vi "Turn Smother.vi"(2 "Ignore Deceleration":bool, 3 "Ignore Acceleration":bool, 4 "input cluster":T5={"Trajectory Data"=[], "Updated Waypoints"=[], "Parameters"={"Sample Period (s)"=0.0, "Limits"={"Velocity (fps)"=6.0, "Accel (fps^2)"=15.0, "Jerk (fps^3)"=150.0, "StoopidFast (fps)"=6.0}, "Conditions"={"vInitial (fps)"=0.0, "vFinal (fps)"=0.0}, "Overrides"=[]}, "Array"=[]} {"Parameters"."Overrides"."Angular Multiplier 2" step=5.0; "Parameters"."Overrides"."Angular Multiplier" step=5.0; "Parameters"."Limits"."StoopidFast (fps)" min=0.0; "Parameters"."Limits"."Jerk (fps^3)" min=0.0 step=1.0; "Parameters"."Limits"."Accel (fps^2)" min=0.0; "Parameters"."Limits"."Velocity (fps)" min=0.0}) -> (1 "Overrides":T1(array[cluster]) {"Angular Multiplier 2" step=5.0; "Angular Multiplier" step=5.0})   [LabVIEW 2019]
uses:
  Types/Limits.ctl
  Types/Single Cmd Info.ctl
  <vilib>/picture/picture.llb/imagedata.ctl
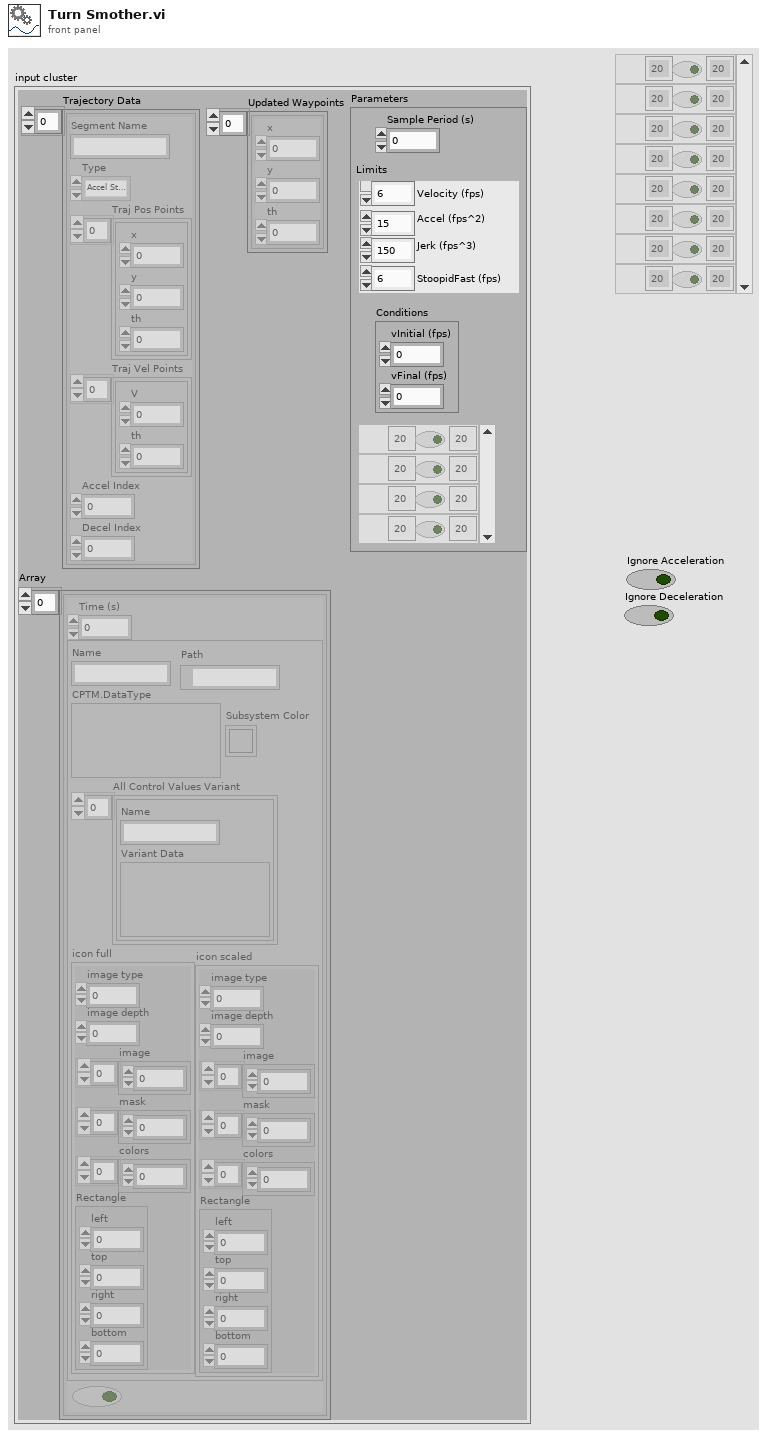
[diagram p1: front panel]
types:
  T1 = cluster{"Count":string, "Angular Multiplier":dbl, "1":bool, "Angular Multiplier 2":dbl}[]
  T2 = typedef "Limits.ctl" = cluster{"Velocity (fps)":dbl, "Accel (fps^2)":dbl, "Jerk (fps^3)":dbl, "StoopidFast (fps)":dbl}
  T3 = typedef "Single Cmd Info.ctl" = cluster{"Name":string, "CPTM.DataType":variant, "All Control Values Variant":cluster{"Name":string, "Variant Data":variant}[], "icon full":T4, "icon scaled":T4, "Path":path, "Subsystem Color":u32}
  T4 = typedef "imagedata.ctl" = cluster{"image type":i32, "image depth":i32, "image":u8[], "mask":u8[], "colors":u32[], "Rectangle":cluster{"left":i16, "top":i16, "right":i16, "bottom":i16}}
  T5 = cluster{"Trajectory Data":cluster{"Segment Name":string, "Type":enum16{"Accel Straight", "Const Straight", "Blend", "Circle"}, "Traj Pos Points":cluster{"x":dbl, "y":dbl, "th":dbl}[], "Traj Vel Points":cluster{"V":dbl, "th":dbl}[], "Accel Index":i32, "Decel Index":i32}[], "Updated Waypoints":cluster{"x":dbl, "y":dbl, "th":dbl}[], "Parameters":cluster{"Sample Period (s)":dbl, "Limits":T2, "Conditions":cluster{"vInitial (fps)":dbl, "vFinal (fps)":dbl}, "Overrides":cluster{"Count":string, "Angular Multiplier":dbl, "1":bool, "Angular Multiplier 2":dbl}[]}, "Array":cluster{"Time (s)":dbl, T3, bool}[]}
  T6 = cluster{"Segment Name":string, "Type":enum16{"Accel Straight", "Const Straight", "Blend", "Circle"}, "Traj Pos Points":cluster{"x":dbl, "y":dbl, "th":dbl}[], "Traj Vel Points":cluster{"V":dbl, "th":dbl}[], "Accel Index":i32, "Decel Index":i32}[]
  T7 = cluster{"Sample Period (s)":dbl, "Limits":T2, "Conditions":cluster{"vInitial (fps)":dbl, "vFinal (fps)":dbl}, "Overrides":cluster{"Count":string, "Angular Multiplier":dbl, "1":bool, "Angular Multiplier 2":dbl}[]}
  T8 = cluster{"vInitial (fps)":dbl, "vFinal (fps)":dbl}
  T9 = cluster{string, dbl, bool, "Velocity (fps)":dbl}[]
  T10 = cluster{"Segment Name":string, "Type":enum16{"Accel Straight", "Const Straight", "Blend", "Circle"}, "Traj Pos Points":cluster{"x":dbl, "y":dbl, "th":dbl}[], "Traj Vel Points":cluster{"V":dbl, "th":dbl}[], "Accel Index":i32, "Decel Index":i32}
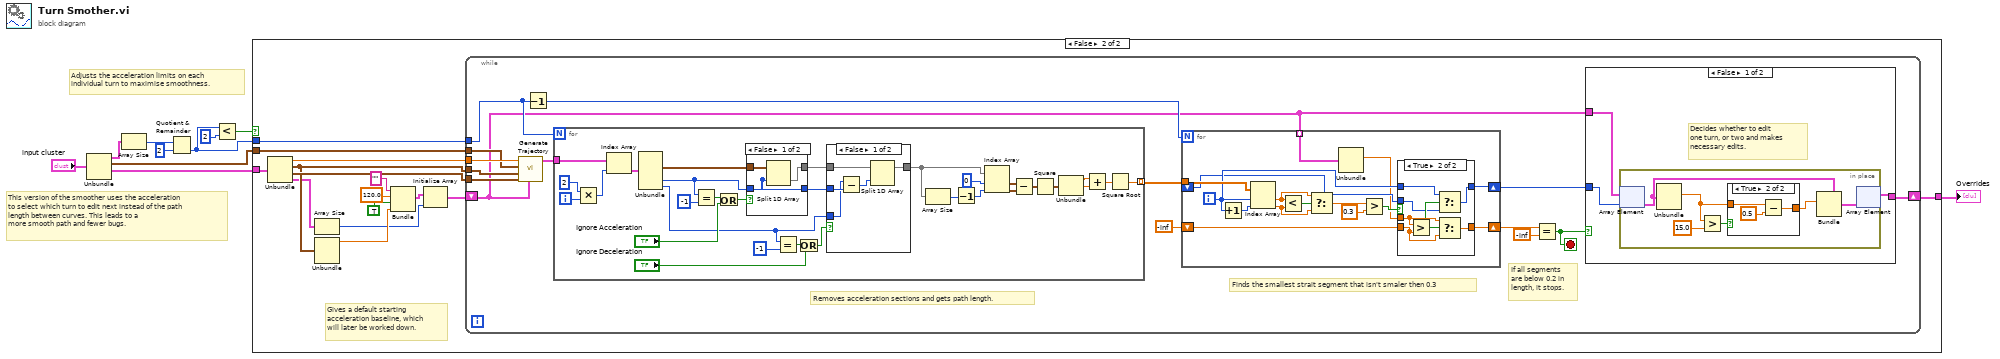
[diagram p0: block diagram]
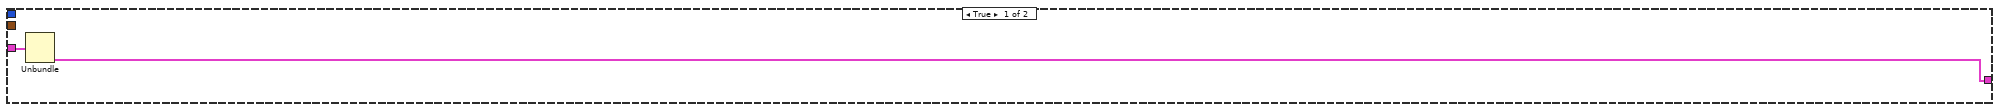
[diagram p2: hidden frame]
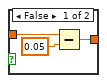
[diagram p3: hidden frame]
diagram:
  # "This version of the smoother uses the acceleration\nto select which turn to edit next instead of the path \nlength between curves. This leads to a \nmore smooth path and fewer bugs."
  # "Adjusts the acceleration limits on each \nindividual turn to maximise smoothness."
  n1 = Unbundle("input cluster") -> ("Trajectory Data"=w3:T6, "Updated Waypoints"=w2:cluster{"x":dbl, "y":dbl, "th":dbl}[], "Parameters"=w4:T7)  [unwired: 1 out]
  n2 = Array Size(array=w3) -> (size(s)=w10:i32)
  n3 = Quotient & Remainder(x=w10, y=2) -> (floor(x/y)=w6:i32)  [unwired: 1 out]
  n4 = Less?(x=w6, y=2) -> (x < y?=w5:bool)
  n5 = case shown="False" w5 {
    tunnel: w6 -> [_ w27]
    tunnel: [w12 w26] -> w1
    tunnel: w4 -> [w11 w25]
    tunnel: w2 -> [_ w23]
    frame True {
      n6 = Unbundle(w11) -> ("Overrides"=w12:T1)  [unwired: 3 out]
    }
    frame False {
      # "Gives a default starting \nacceleration baseline, which\nwill later be worked down."
      n7 = Unbundle(w25) -> ("Sample Period (s)"=w24:dbl, "Limits"=w21:T2, "Conditions"=w22:T8, "Overrides"=w20:T1)
      n8 = Array Size(array=w20) -> (size(s)=w15:i32)
      n9 = Unbundle(w21) -> ("Velocity (fps)"=w16:dbl)  [unwired: 3 out]
      n10 = Bundle("", 120.0, TRUE, "Velocity (fps)"=w16) -> (w14:cluster{string, dbl, bool, "Velocity (fps)":dbl})  [unwired: 1 in]
      n11 = Initialize Array(w14, w15) -> (w13:T9)
      n12 = while {
        shift-right: [w40] -> w26
        shift-left: w13 -> [w28]
        tunnel: w27 -> [w37]
        tunnel: w24 -> [w35]
        tunnel: w23 -> [w34]
        tunnel: w21 -> [w33]
        tunnel: w22 -> [w32]
        stop <- w42 stop-if-true
        # "If all segments\nare below 0.2 in\nlength, it stops."
        # "Removes acceleration sections and gets path length."
        # "Finds the smallest strait segment that isn't smaler then 0.3"
        n13 = call "Generate Trajectory.vi"("Overrides 2"=w28, "Conditions"=w32, "Limits"=w33, "WayPoints"=w34, "Sample Period (s)"=w35) -> ("Trajectory Data"=w36:T6)  [unwired: 2 in, 4 out]
        n14 = Decrement(x=w37) -> (x-1=w38:i32)
        n15 = for {
          N: w37 -> [_]
          tunnel: w36 -> [w86]
          tunnel: [w76] -> w39 mode=indexing
          i -> [w88]
          n16 = Multiply(x=2, y=w88) -> (x*y=w85:i32)
          n17 = Index Array(array=w86, index=w85) -> (element=w84:T10)
          n18 = Unbundle(w84) -> ("Traj Pos Points"=w77:cluster{"x":dbl, "y":dbl, "th":dbl}[], "Accel Index"=w73:i32, "Decel Index"=w66:i32)  [unwired: 3 out]
          n19 = Equal?(x=w73, y=-1) -> (x = y?=w74:bool)
          n20 = Or(x=w74, y="Ignore Acceleration") -> (x .or. y?=w72:bool)
          n21 = case shown="False" w72 {
            tunnel: w77 -> [w97 w98]
            tunnel: [w96 w98] -> w83
            tunnel: [w95 _] -> w82
            tunnel: w73 -> [w95 _]
            frame False {
              n22 = Split 1D Array(array=w97, index=w95) -> (second subarray=w96:cluster{"x":dbl, "y":dbl, "th":dbl}[])  [unwired: 1 out]
            }
            frame True {
            }
          }
          n23 = Equal?(x=w66, y=-1) -> (x = y?=w69:bool)
          n24 = Or(x=w69, y="Ignore Deceleration") -> (x .or. y?=w67:bool)
          n25 = case shown="False" w67 {
            tunnel: w83 -> [w93 w94]
            tunnel: [w92 w94] -> w80
            tunnel: w82 -> [w91 _]
            tunnel: w66 -> [w89 _]
            frame False {
              n26 = Subtract(x=w89, y=w91) -> (x-y=w90:i32)
              n27 = Split 1D Array(array=w93, index=w90) -> (first subarray=w92:cluster{"x":dbl, "y":dbl, "th":dbl}[])  [unwired: 1 out]
            }
            frame True {
            }
          }
          n28 = Array Size(array=w80) -> (size(s)=w79:i32)
          n29 = Decrement(x=w79) -> (x-1=w78:i32)
          n30 = Index Array(array=w80, index #1=0 ("index"), index #2=w78) -> (element #1=w65:cluster{"x":dbl, "y":dbl, "th":dbl}, element #2=w64:cluster{"x":dbl, "y":dbl, "th":dbl})
          n31 = Subtract(x=w65, y=w64) -> (x-y=w63:cluster{"x":dbl, "y":dbl, "th":dbl})
          n32 = Square(x=w63) -> (x^2=w62:cluster{"x":dbl, "y":dbl, "th":dbl})
          n33 = Unbundle(w62) -> ("x"=w60:dbl, "y"=w61:dbl)  [unwired: 1 out]
          n34 = Add(x=w60, y=w61) -> (x+y=w59:dbl)
          n35 = Square Root(x=w59) -> (sqrt(x)=w76:dbl)
        }
        n36 = for {
          N: w38 -> [_]
          tunnel: w39 -> [w113]
          shift-right: [w108] -> w41
          shift-left: -inf -> [w107]
          tunnel: w28 -> [w100] mode=indexing
          shift-right: [w102] -> w29
          shift-left: _ -> [w101]
          i -> [w103]
          n37 = Increment(x=w103) -> (x+1=w112:i32)
          n38 = Index Array(array=w113, index #1=w103, index #2=w112) -> (element #1=w109:dbl, element #2=w110:dbl)
          n39 = Less?(x=w109, y=w110) -> (x < y?=w111:bool)
          n40 = Select(t=w109, s=w111, f=w110) -> (s? t:f=w105:dbl)
          n41 = Unbundle(w100) -> (w99:dbl)  [unwired: 3 out]
          n42 = Greater?(x=w105, y=0.3) -> (0:w106:bool)
          n43 = case shown="True" w106 {
            tunnel: [w115 w122] -> w108
            tunnel: w107 -> [w115 w121]
            tunnel: w99 -> [_ w120]
            tunnel: w103 -> [_ w118]
            tunnel: [w114 w116] -> w102
            tunnel: w101 -> [w114 w117]
            frame False {
            }
            frame True {
              n44 = Greater?(x=w120, y=w121) -> (0:w119:bool)
              n45 = Select(t=w118, s=w119, f=w117) -> (s? t:f=w116:i32)
              n46 = Select(t=w120, s=w119, f=w121) -> (s? t:f=w122:dbl)
            }
          }
        }
        n47 = Equal?(x=w41, y=-inf) -> (x = y?=w42:bool)
        n48 = case shown="False" w42 {
          tunnel: w28 -> [w43 w58]
          tunnel: [w44 w58] -> w40
          tunnel: w29 -> [w45 _]
          frame False {
            # "Decides whether to edit\none turn, or two and makes\nnecessary edits."
            n49 = in-place {
              n50 = in-place-array #1(w43, w45) -> (w48:cluster{string, dbl, bool, "Velocity (fps)":dbl})
              n51 = Unbundle(w48) -> (w49:dbl)  [unwired: 3 out]
              n52 = Greater?(x=w49, y=15.0) -> (0:w50:bool)
              n53 = case shown="True" w50 {
                tunnel: [w53 w56] -> w47
                tunnel: w49 -> [w54 w55]
                frame False {
                  n54 = Subtract(x=w54, y=0.05) -> (x-y=w53:dbl)
                }
                frame True {
                  n55 = Subtract(x=w55, y=0.5) -> (x-y=w56:dbl)
                }
              }
              n56 = Bundle(cluster=w48, w47) -> (w46:cluster{string, dbl, bool, "Velocity (fps)":dbl})  [unwired: 3 in]
              n57 = in-place-array #1(w46) -> (w44:T9)  [unwired: 1 out]
            }
          }
          frame True {
          }
        }
      }
    }
  }
  "Overrides" <- w1
